vi "Generate Waveforms.vi"(6 "reset phase":bool, 8 "error in (no error)":errorcluster, 11 "Generator.lvclass":refnum<class "Generator.lvclass">) -> (0 "error out":errorcluster, 1 "Chart":dbl(graph), 2 "Waveforms out":T7, 3 "Generator.lvclass":refnum<class "Generator.lvclass">, 4 "phase reset":bool)   [LabVIEW 2019, in "Generator.lvclass"]
uses:
  Generator.lvclass
  typedefs/Waveforms--Cluster.ctl
  typedefs/Generator.Sweep State--enum.ctl
  typedefs/Sampling--Cluster.ctl
  typedefs/AO.Channel.Function--Enum.ctl
  typedefs/AO.Channel--Cluster.ctl
  typedefs/AO.Channel--Cluster--Array.ctl
  typedefs/REF.Channel--Cluster.ctl
  typedefs/REF.Channel--Cluster--Array.ctl
panel:
  out "configuration.REF Channels":T1
  out "configuration.AO Channels":T3
  out "configuration.Sampling":T6
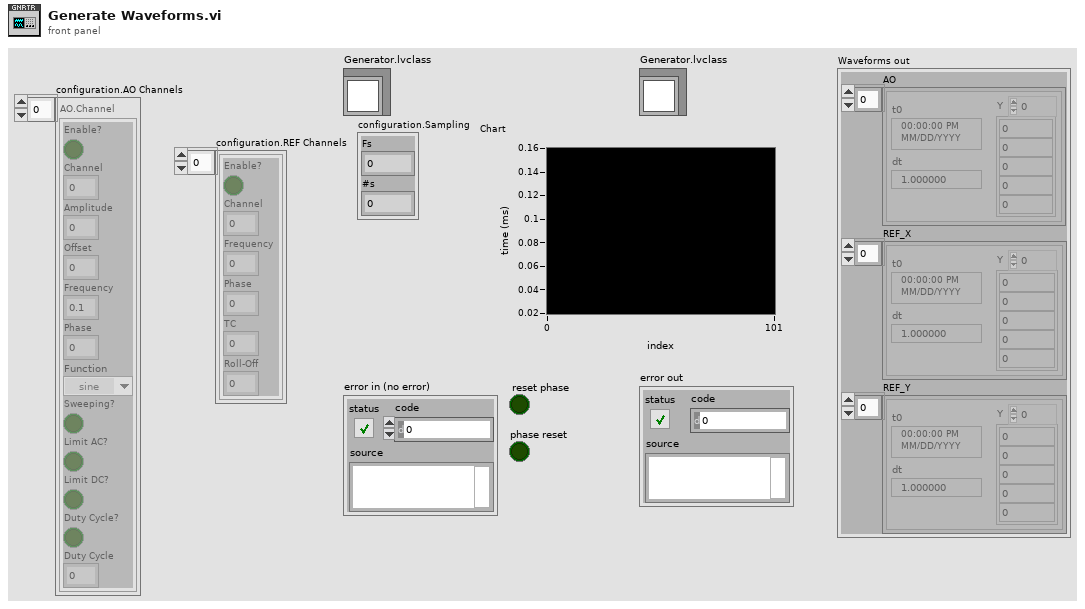
[diagram p1: front panel]
types:
  T1 = typedef "Generator.lvclass/REF.Channel--Cluster--Array.ctl" = T2[]
  T2 = typedef "Generator.lvclass/REF.Channel--Cluster.ctl" = cluster{"Enable?":bool, "Channel":i32, "Frequency":dbl, "Phase":dbl, "TC":dbl, "Roll-Off":i32}
  T3 = typedef "Generator.lvclass/AO.Channel--Cluster--Array.ctl" = T4[]
  T4 = typedef "Generator.lvclass/AO.Channel--Cluster.ctl" = cluster{"Enable?":bool, "Channel":i32, "Amplitude":dbl, "Offset":dbl, "Frequency":dbl, "Phase":dbl, "Function":T5, "Sweeping?":bool, "Limit AC?":bool, "Limit DC?":bool, "Duty Cycle?":bool, "Duty Cycle":dbl}
  T5 = typedef "Generator.lvclass/AO.Channel.Function--Enum.ctl" = enum16{"sine", "square", "triangle", "saw"}
  T6 = typedef "Generator.lvclass/Sampling--Cluster.ctl" = cluster{"Fs":dbl, "#s":dbl}
  T7 = typedef "Generator.lvclass/Waveforms--Cluster.ctl" = cluster{"AO":waveform(dbl)[], "REF_X":waveform(dbl)[], "REF_Y":waveform(dbl)[]}
  T8 = typedef "Generator.lvclass/Generator.Sweep State--enum.ctl" = enum16{"idle", "initialize", "wait", "sweep", "stop"}
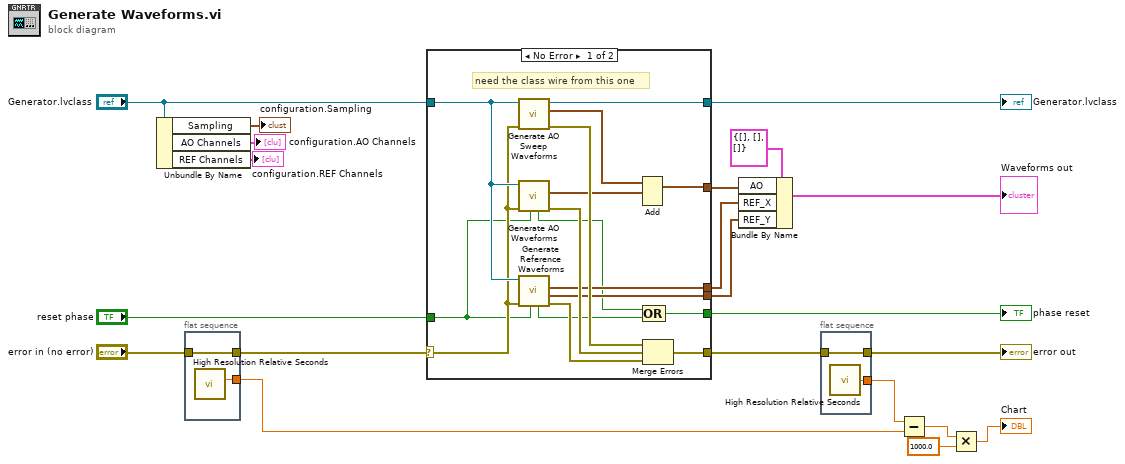
[diagram p0: block diagram]
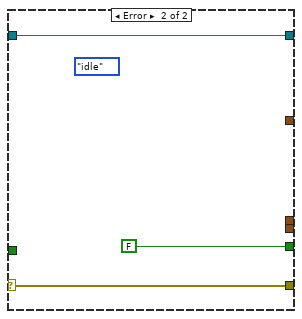
[diagram p2: hidden frame]
diagram:
  n1 = Unbundle By Name("Generator.lvclass") -> ("Sampling"=→"configuration.Sampling":T6, "AO Channels"=→"configuration.AO Channels":T3, "REF Channels"=→"configuration.REF Channels":T1)
  n2 = flat-sequence {
    tunnel: [w23] -> w8
    tunnel: "error in (no error)" -> [w22]
    tunnel: [w22] -> w11
    frame #0 {
      n3 = call <vilib>:"High Resolution Relative Seconds.vi"() -> ("relative seconds"=w23:dbl)
    }
  }
  n4 = case shown="No Error" w11 {
    selector: w11 -> [w25 w42]
    tunnel: [w33 _] -> w17
    tunnel: [w34 _] -> w19
    tunnel: [w39 w42] -> w10
    tunnel: "Generator.lvclass" -> [w26 w41]
    tunnel: [w37 w41] -> w16
    tunnel: [w32 _] -> w18
    tunnel: [w27 FALSE] -> w15
    tunnel: "reset phase" -> [w24 _]
    frame No Error {
      # "need the class wire from this one"
      n5 = call "Generate AO Sweep Waveforms.vi"("error in (no error)"=w25, "Generator"=w26) -> ("error out"=w35:errorcluster, "AO Array"=w31:waveform(dbl)[], "Generator out"=w37:refnum<class "Generator.lvclass">)  [unwired: 7 in]
      n6 = call "Generate AO Waveforms.vi"("reset phase"=w24, "error in (no error)"=w25, "Generator in"=w26) -> ("error out"=w36:errorcluster, "AO Array"=w30:waveform(dbl)[], "phase reset"=w28:bool)  [unwired: 5 in, 1 out]
      n7 = call "Generate Reference Waveforms.vi"("reset phase"=w24, "error in (no error)"=w25, "Generator in"=w26) -> ("error out"=w38:errorcluster, "REF_Y"=w32:waveform(dbl)[], "REF_X"=w33:waveform(dbl)[], "phase reset"=w29:bool)  [unwired: 4 in, 1 out]
      n8 = Add(1:w30, 2:w31) -> (0:w34:waveform(dbl)[])  [unwired: 1 in, 1 out]
      n9 = Compound Arithmetic op=OR(w28, w29) -> (w27:bool)
      n10 = Merge Errors(w35, w36, w38) -> (w39:errorcluster)
    }
    frame Error {
      (unwired) Generator.Sweep_State--enum."idle" ("sweep state out")
    }
  }
  "Generator.lvclass" <- w16
  "phase reset" <- w15
  n11 = Bundle By Name(cluster=T7 {"AO"=[], "REF_X"=[], "REF_Y"=[]} ("Waveforms"), "AO"=w19, "REF_X"=w17, "REF_Y"=w18) -> (→"Waveforms out":T7)
  n12 = flat-sequence {
    tunnel: [w44] -> w13
    tunnel: w10 -> [w43]
    tunnel: [w43] -> w9
    frame #0 {
      n13 = call <vilib>:"High Resolution Relative Seconds.vi"() -> ("relative seconds"=w44:dbl)
    }
  }
  n14 = Subtract(x=w13, y=w8) -> (x-y=w6:dbl)
  n15 = Multiply(x=w6, y=1000.0) -> (x*y=→"Chart":dbl)
  "error out" <- w9
